vi "Test_Destroy.vi"(8 "error in (no error)":errorcluster, 11 "TestCase in":refnum<class "List_Delegations.lvclass">) -> (0 "error out":errorcluster, 3 "TestCase out":refnum<class "List_Delegations.lvclass">)   [LabVIEW 2009, in "List_Delegations.lvclass"]
uses:
  List_Delegations.lvclass
  List_Delegations.lvclass/List_Delegations.ctl
  source/Lists/List/List.lvclass
  Test Doubles/ListImp_RefSpy/ListImp_RefSpy.lvclass
  UnitTestComparisons/UnitTestComparisons.lvlib
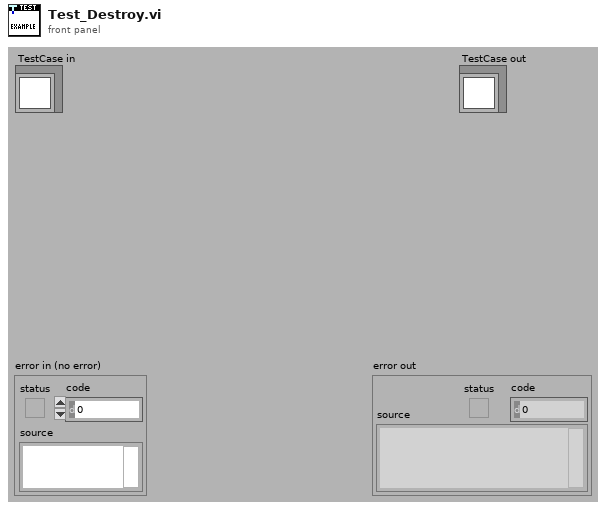
[diagram p1: front panel]
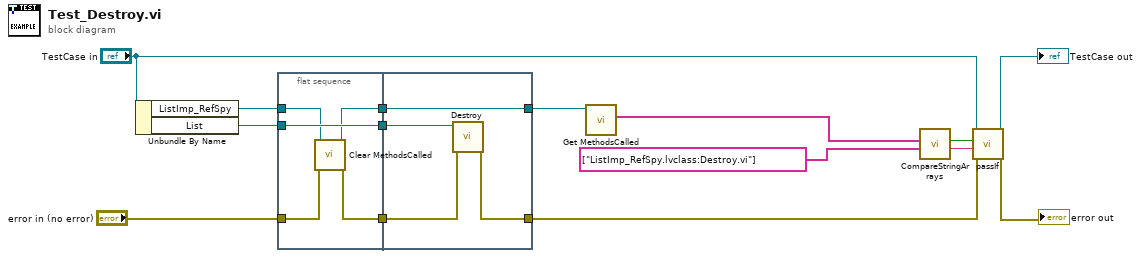
[diagram p0: block diagram]
diagram:
  n1 = Unbundle By Name("TestCase in") -> ("ListImp_RefSpy"=w10:refnum<class "ListImp_RefSpy.lvclass">, "List"=w12:refnum<class "List.lvclass">)
  n2 = flat-sequence {
    tunnel: w10 -> [w19]
    tunnel: "error in (no error)" -> [w17]
    tunnel: w12 -> [w20]
    tunnel: [w20] -> w9
    tunnel: [w16] -> w8
    tunnel: [w18] -> w7
    tunnel: w9 -> [w24]
    tunnel: w8 -> [w22]
    tunnel: w7 -> [w21]
    tunnel: [w23] -> w5
    tunnel: [w21] -> w6
    frame #0 {
      n3 = call "Clear MethodsCalled.vi"("error in (no error)"=w17, "MockListImp in"=w19) -> ("error out"=w16:errorcluster, "MockListImp out"=w18:refnum<class "ListImp_RefSpy.lvclass">)  [unwired: 8 in]
    }
    frame #1 {
      n4 = call-dynamic "Destroy.vi"("error in (no error)"=w22, "List in"=w24) -> ("error out"=w23:errorcluster)  [unwired: 9 in]
    }
  }
  n5 = call "Get MethodsCalled.vi"("MockListImp"=w6) -> ("MethodsCalled"=w4:string[])  [unwired: 9 in, 1 out]
  n6 = call "CompareStringArrays.vi"("Expected Strings"=string[] ["ListImp_RefSpy.lvclass:Destroy.vi"] ("MethodsCalled"), "Actual Strings"=w4) -> ("Message"=w1:string, "Equal?"=w2:bool)  [unwired: 8 in]
  n7 = call-dynamic "passIf.vi"("error in (no error)"=w5, "message (\"\")"=w1, "pass"=w2, "TestCase in"="TestCase in") -> ("error out"=→"error out":errorcluster, "TestCase out"=→"TestCase out":refnum<class "List_Delegations.lvclass">)  [unwired: 6 in]
